vi "CMC-InClass-Simple Tank Model.vi"() -> ()   [LabVIEW 2010]
panel:
  out "Tank Volume (liters):":dbl format="%#.2g"
  out "Tank (gal)":dbl(slide) scale=0.0..22.0
  in  "Tank Volume (gal)":dbl(knob) min=0.0 max=19.0 scale=0.0..19.0 scale format="%#_2g"
  # "MY NAME IS: CLAIR CUNNINGHAM"
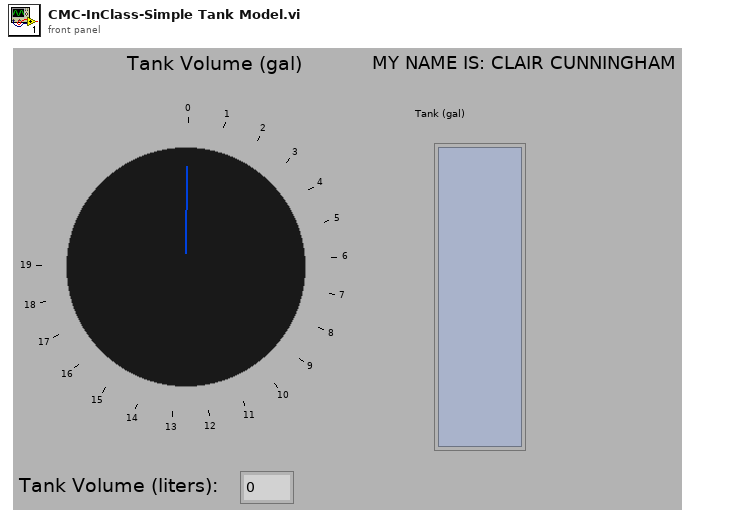
[diagram p1: front panel]
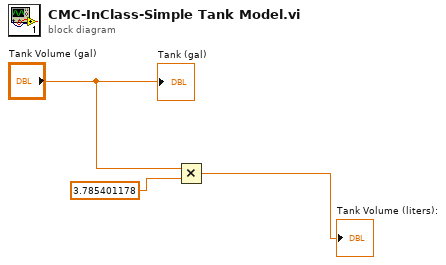
[diagram p0: block diagram]
diagram:
  n1 = Multiply(x="Tank Volume (gal)", y=3.785401178) -> (x*y=→"Tank Volume (liters):":dbl)
  "Tank (gal)" <- "Tank Volume (gal)"
